vi "InjectApplicationReference.vi"(8 "error in (no error)":errorcluster, 10 "Application":refnum<vi>, 11 "CreateInterface in":refnum<class "CreateInterface.lvclass">) -> (0 "error out":errorcluster, 3 "CreateInterface out":refnum<class "CreateInterface.lvclass">)   [LabVIEW 2020, in "Mermaid.lvlib" / "CreateInterface.lvclass"]
uses:
  CreateInterface.lvclass
  CreateInterface.lvclass/CreateInterface.ctl
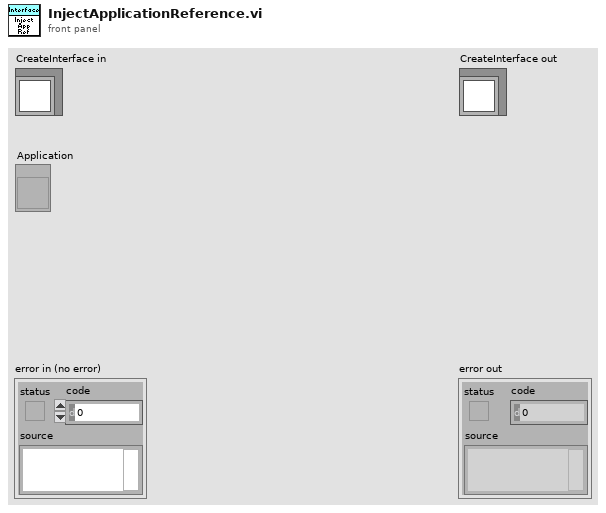
[diagram p1: front panel]
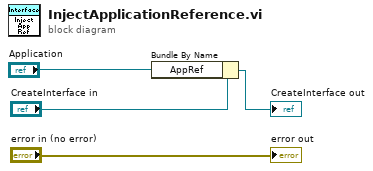
[diagram p0: block diagram]
diagram:
  n1 = Bundle By Name(cluster="CreateInterface in", "AppRef"="Application") -> (→"CreateInterface out":refnum<class "CreateInterface.lvclass">)
  "error out" <- "error in (no error)"
